vi "Calculator.vi"(8 "error in (no error)":errorcluster, 9 "Operation":T1, 10 "b":dbl, 11 "a":dbl) -> (0 "error out":errorcluster, 3 "result":dbl)   [LabVIEW 2018]
uses:
  Operation_control.ctl
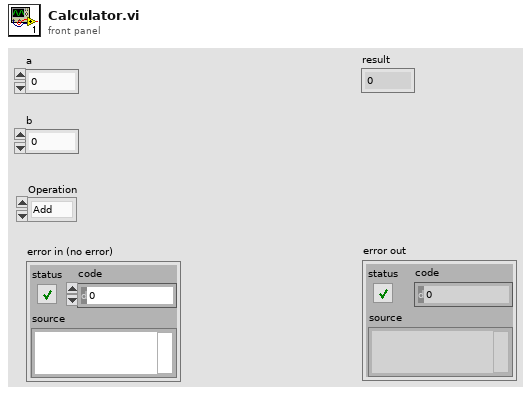
[diagram p1: front panel]
types:
  T1 = typedef "Operation_control.ctl" = enum16{"Add", "Subtract", "Multiply", "Divide"}
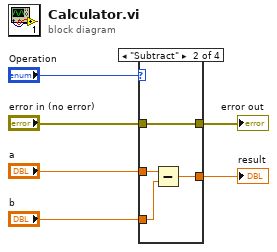
[diagram p0: block diagram]
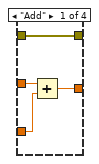
[diagram p2: hidden frame]
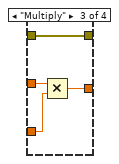
[diagram p3: hidden frame]
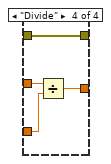
[diagram p4: hidden frame]
diagram:
  n1 = case shown="\"Subtract\"" "Operation" {
    tunnel: [w10 w14 w18 w19] -> w2
    tunnel: "error in (no error)" -> [w10 w14 w18 w19]
    tunnel: "a" -> [w9 w13 w17 w22]
    tunnel: "b" -> [w8 w12 w16 w20]
    tunnel: [w7 w11 w15 w21] -> w3
    frame "Add" {
      n2 = Add(x=w9, y=w8) -> (x+y=w7:dbl)
    }
    frame "Subtract" {
      n3 = Subtract(x=w13, y=w12) -> (x-y=w11:dbl)
    }
    frame "Multiply" {
      n4 = Multiply(x=w17, y=w16) -> (x*y=w15:dbl)
    }
    frame "Divide" {
      n5 = Divide(x=w22, y=w20) -> (x/y=w21:dbl)
    }
  }
  "result" <- w3
  "error out" <- w2
